vi "onTestExecution.vi"(7 "Name":string, 8 "error in (no error)":errorcluster, 11 "Unit Tests for Runner in":refnum<class "Unit Tests for Runner.lvclass">) -> (0 "error out":errorcluster, 3 "Unit Tests for Runner out":refnum<class "Unit Tests for Runner.lvclass">)   [LabVIEW 2013, in "Unit Tests for Runner.lvclass"]
uses:
  Unit Tests for Runner.lvclass
  classes/Test Runner/Test Runner.lvclass
  classes/Test/Test.lvclass
  classes/Assert/Assert.lvclass
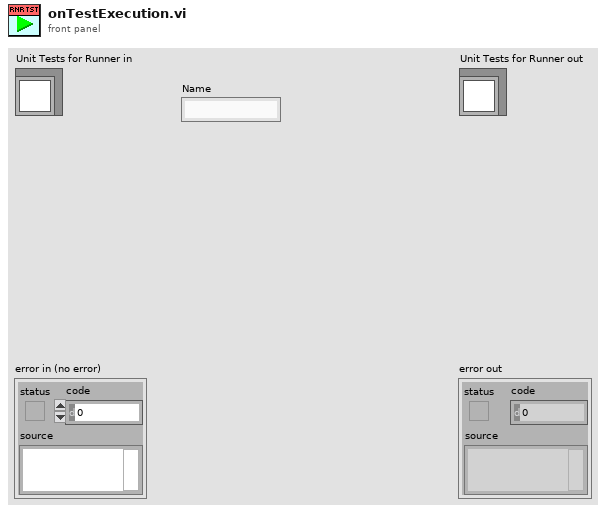
[diagram p1: front panel]
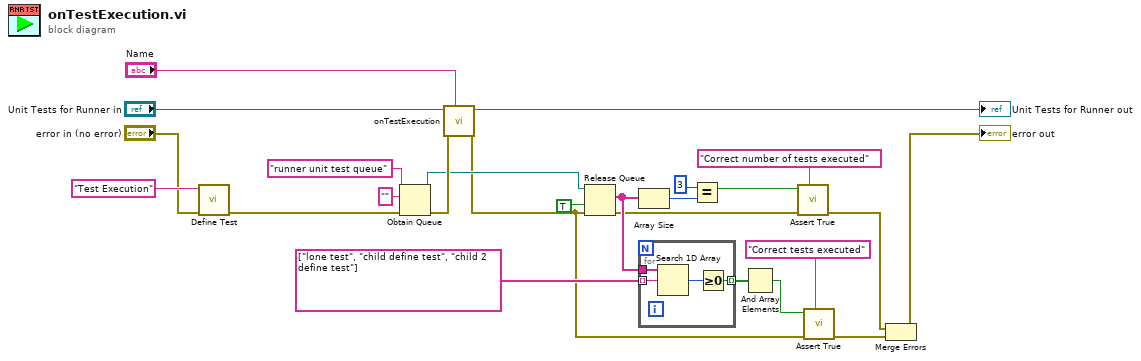
[diagram p0: block diagram]
diagram:
  n1 = call "Define Test.vi"("error in (no error)"="error in (no error)", "Label (VI Title)"="Test Execution" ("name (unnamed)")) -> ("error out"=w1:errorcluster)  [unwired: 9 in]
  n2 = Obtain Queue(name (unnamed)="runner unit test queue", element data type="", error in (no error)=w1) -> (queue out=w6:refnum<queue>, error out=w20:errorcluster)  [unwired: 2 in, 1 out]
  n3 = call-parent "onTestExecution.vi"("Name"="Name", "error in (no error)"=w20, "Test Runner in"="Unit Tests for Runner in") -> ("error out"=w3:errorcluster, "Test Runner out"=→"Unit Tests for Runner out":refnum<class "Unit Tests for Runner.lvclass">)  [unwired: 7 in]
  n4 = Release Queue(queue=w6, force destroy? (F)=TRUE, error in (no error)=w3) -> (remaining elements=w17:string[], error out=w13:errorcluster)  [unwired: 1 out]
  n5 = Array Size(array=w17) -> (size(s)=w16:i32)
  n6 = for {
    tunnel: w17 -> [w29]
    tunnel: string[] ["lone test", "child define test", "child 2 define test"] -> [w28] mode=indexing
    tunnel: [w26] -> w12 mode=indexing
    n7 = Search 1D Array(1D array=w29, element=w28) -> (index of element=w27:i32)  [unwired: 1 in]
    n8 = Greater Or Equal To 0?(x=w27) -> (x >= 0?=w26:bool)
  }
  n9 = Equal?(x=3, y=w16) -> (x = y?=w8:bool)
  n10 = And Array Elements(Boolean array=w12) -> (logical AND=w9:bool)
  n11 = call "Assert True.vi"("Label"="Correct number of tests executed", "error in (no error)"=w13, "True?"=w8) -> ("error out"=w7:errorcluster)  [unwired: 8 in]
  n12 = call "Assert True.vi"("Label"="Correct tests executed", "error in (no error)"=w3, "True?"=w9) -> ("error out"=w10:errorcluster)  [unwired: 8 in]
  n13 = Merge Errors(w7, w10) -> (→"error out":errorcluster)
